vi "Pert_MotorSelect3D.vi"(4 "Pert Direction":i16, 6 "y_Fdesired":dbl, 7 "condition":bool) -> (2 "DesTensions":dbl[](array[numeric]))   [LabVIEW 2017]
uses:
  <vilib>/imath/engines/lvmath2/RunTimeEngine/Managers/WorkSpace/UID Generator.vi
  <vilib>/imath/engines/lvmath2/RunTimeEngine/IndexRead/NIMS M(S).vi
  <instcachedir>/0/NIMS M(S)_B826C018497E4940AE96BD27B540B6FB.lvgen/NIMS M(S)_B826C018497E4940AE96BD27B540B6FB_000.vi
  <vilib>/imath/engines/lvmath2/RunTimeEngine/ErrorHandling/NIMS_Create Error From Enums.vi
  <vilib>/imath/engines/lvmath2/RunTimeEngine/IndexRead/NIMS V(S).vi
  <instcachedir>/0/NIMS V(S)_0488751826AF41519A22953C041130DC.lvgen/NIMS V(S)_0488751826AF41519A22953C041130DC_000.vi
  <vilib>/imath/engines/lvmath2/RunTimeEngine/RunTimeType/NIMS_RunTimeType_From StrictType (excl LVString).vi
  <instcachedir>/0/NIMS_RunTimeType_From StrictType (excl LVString)_1019F277F0A747EDBCA0F6C52CA54500.lvgen/NIMS_RunTimeType_From StrictType (excl LVString)_1019F277F0A747EDBCA0F6C52CA54500_000.vi
  <vilib>/imath/engines/lvmath2/RunTimeEngine/LocalVariableDefStatement/MC_LocalVariableDefStatement_Display.vi
  <vilib>/imath/engines/lvmath2/RunTimeEngine/BuiltInFunctions/sin/NIMS_sin(C).vi
  <instcachedir>/0/NIMS_sin(C)_3AEF00A0D47841AA8A3F5FC7392BEEFD.lvgen/NIMS_sin(C)_3AEF00A0D47841AA8A3F5FC7392BEEFD_001.vi
  <vilib>/imath/engines/lvmath2/RunTimeEngine/BuiltInFunctions/cos/NIMS_cos(C).vi
  <instcachedir>/0/NIMS_cos(C)_D76AB42705D04DD7AB90183D51B32C21.lvgen/NIMS_cos(C)_D76AB42705D04DD7AB90183D51B32C21_001.vi
  <vilib>/imath/engines/lvmath2/RunTimeEngine/VariableToken/NIMS_VariableToken_CondDefined.vi
  <instcachedir>/0/NIMS_VariableToken_CondDefined_6E7F1EE7F80E48298C84CF05BD736261.lvgen/NIMS_VariableToken_CondDefined_6E7F1EE7F80E48298C84CF05BD736261_000.vi
  <vilib>/imathl/engines/lvmath/Functions/Error Handling/Create Error.vi
  <vilib>/imath/engines/lvmath2/RunTimeEngine/Managers/SymbolTable/Clear UID.vi
  <vilib>/imath/engines/lvmath2/RunTimeEngine/NodeEndStatement/NIMS_NodeEndStatement_Output.vi
  <instcachedir>/0/NIMS_NodeEndStatement_Output_53EC0D466D134D7ABD903AC30B43404B.lvgen/NIMS_NodeEndStatement_Output_53EC0D466D134D7ABD903AC30B43404B_000.vi
  <vilib>/imath/engines/lvmath2/RunTimeEngine/ErrorHandling/NIMS_Finalize Error.vi
  <vilib>/imath/engines/lvmath2/RunTimeEngine/Managers/SymbolTable/NIMS_WorkSpace.lvlib
panel:
  # "3D Pelvic Perturbations"
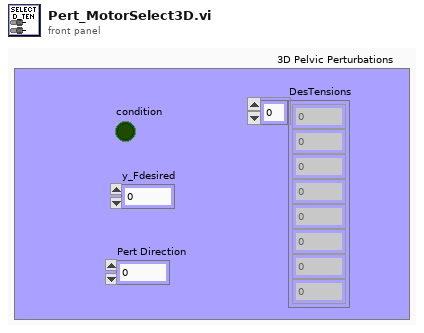
[diagram p1: front panel]
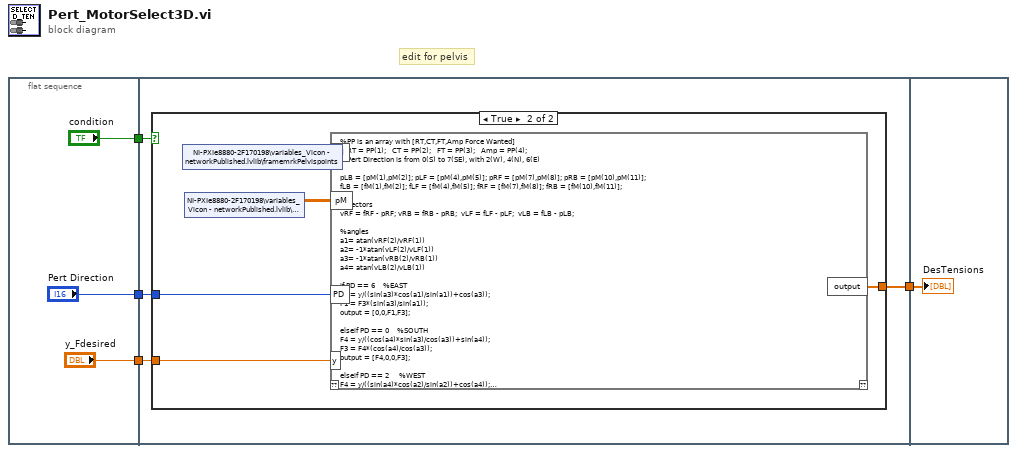
[diagram p0: block diagram]
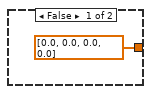
[diagram p2: hidden frame]
diagram:
  # "edit for pelvis"
  n1 = flat-sequence {
    tunnel: ["condition"] -> w4
    tunnel: ["y_Fdesired"] -> w2
    tunnel: ["Pert Direction"] -> w1
    tunnel: w4 -> [w11]
    tunnel: [w8] -> w3
    tunnel: w2 -> [w10]
    tunnel: w1 -> [w9]
    tunnel: w3 -> [w848]
    frame #0 {
    }
    frame #1 {
      n2 = case shown="True" w11 {
        tunnel: [dbl[] [0.0, 0.0, 0.0, 0.0] w15] -> w8
        tunnel: w10 -> [_ w14]
        tunnel: w9 -> [_ w13]
        frame False {
        }
        frame True {
          n3 = shared-variable "NI-PXIe8880-2F170198\\variables_Vicon - networkPublished.lvlib\\framemrkPelvispoints"() -> (w17:dbl[][])  [unwired: 1 in, 1 out]
          n4 = shared-variable "NI-PXIe8880-2F170198\\variables_Vicon - networkPublished.lvlib\\braceptsPelvis"() -> (w16:dbl[][])  [unwired: 1 in, 1 out]
          n5 = mathscript code="%PP is an array with [RT,CT,FT,Amp Force Wanted]\n%RT = PP(1);   CT = PP(2);   FT = PP(3);   Amp = PP(4);\n%Pert Direction is from 0(S) to 7(SE), with 2(W), 4(N), 6(E)\n\npLB = [pM(1),pM(2)]; pLF = [pM(4),pM(5)]; pRF = [pM(7),pM(8)]; pRB = [pM(10),pM(11)];\nfLB = [fM(1),fM(2)]; fLF = [fM(4),fM(5)]; fRF = [fM(7),fM(8)]; fRB = [fM(10),fM(11)];\n\n%vectors\nvRF = fRF - pRF; vRB = fRB - pRB;  vLF = fLF - pLF;  vLB = fLB - pLB; \n\n%angles\na1= atan(vRF(2)/vRF(1))\na2= -1*atan(vLF(2)/vLF(1))\na3= -1*atan(vRB(2)/vRB(1))\na4= atan(vLB(2)/vLB(1))\n\nif PD == 6    %EAST \nF3 = y/((sin(a3)*cos(a1)/sin(a1))+cos(a3));\nF1 = F3*(sin(a3)/sin(a1));\noutput = [0,0,F1,F3];\n\nelseif PD == 0    %SOUTH\nF4 = y/((cos(a4)*sin(a3)/cos(a3))+sin(a4));\nF3 = F4*(cos(a4)/cos(a3));\noutput = [F4,0,0,F3];\n\nelseif PD == 2     %WEST\nF4 = y/((sin(a4)*cos(a2)/sin(a2))+cos(a4));\nF2 = F4*(sin(a4)/sin(a2));\noutput = [F4,F2,0,0];\n\nelseif PD == 4    %NORTH\nF2 = y/((cos(a2)*sin(a1)/cos(a1))+sin(a2));\nF1 = F2*(cos(a2)/cos(a1));\noutput = [0,F2,F1,0];\n\nelseif PD == 1\noutput = [y,0,0,0]\n\nelseif PD == 3\noutput = [0,y,0,0]\n\nelseif PD == 5\noutput = [0,0,y,0]\n\nelseif PD == 7\noutput = [0,0,0,y]\nend"("fM"=w17, "pM"=w16, "PD"=w13, "y"=w14) -> ("output"=w15:cdb[])  [unwired: 1 in, 1 out]
        }
      }
    }
    frame #2 {
      "DesTensions" <- w848
    }
  }
